vi "Create.vi"(10 "Events Summary":T1) -> (3 "Events Summary Value out":refnum<class "Events Summary Value.lvclass">)   [LabVIEW 2020, in "Volatus.lvlib" / "Events Summary Value.lvclass"]
uses:
  Events Summary Value.lvclass
  Events Summary Value.lvclass/Events Summary Value.ctl
  Events Summary.ctl
  Volatus.lvlib
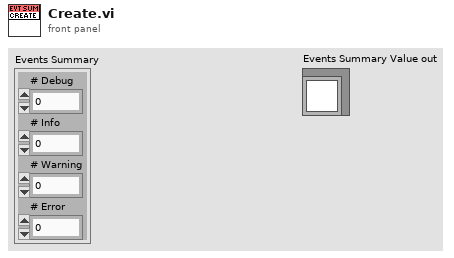
[diagram p1: front panel]
types:
  T1 = typedef "Volatus.lvlib/Events Summary.ctl" = cluster{"# Debug":i32, "# Info":i32, "# Warning":i32, "# Error":i32}
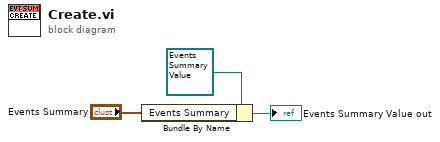
[diagram p0: block diagram]
diagram:
  n1 = Bundle By Name(cluster=refnum<class "Events Summary Value.lvclass"> refnum ("Events Summary Value in"), "Events Summary"="Events Summary") -> (→"Events Summary Value out":refnum<class "Events Summary Value.lvclass">)
